vi "Save_dialogue_Q.vi"(5 "Номер образца":i32, 7 "Интеграл":dbl, 8 "0 level":bool, 9 "1 level":bool, 10 "Мощность":dbl, 11 "Амплитуда":dbl) -> (0 "OK Button 2":bool, 1 "stop 2":bool, 2 "Название 2":string, 3 "Путь 2":path)   [LabVIEW 2013]
panel:
  in  "Путь к файлу 0 уровень":path=path "d:/mech/LVPROG/1642RK2U_2port/Oscillograms/0 Level"
  in  "Путь к файлу 1 уровень":path=path "d:/mech/LVPROG/1642RK2U_2port/Oscillograms/1 Level"
  in  "Номер образца":string="1"
  in  "stop":bool
  in  "OK Button":bool
  in  "Мощность дозы":string="0,0E+0"
  in  "Путь к файлу имп.реакций":path=path "d:/mech/LVPROG/1642RK2U_2port/Oscillograms/Imp_reaction"
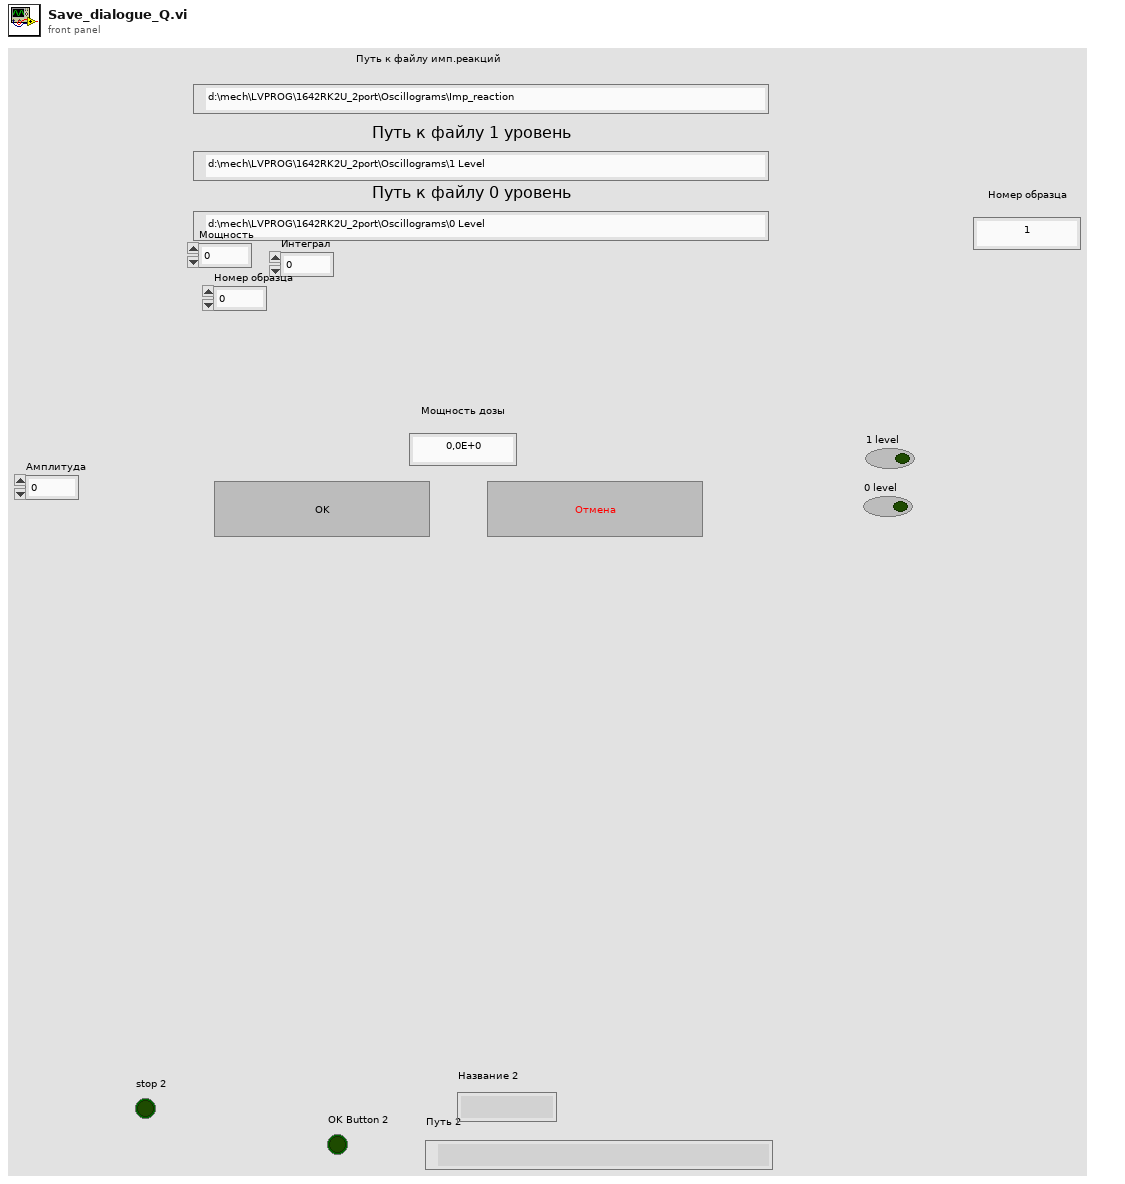
[diagram p1: front panel]
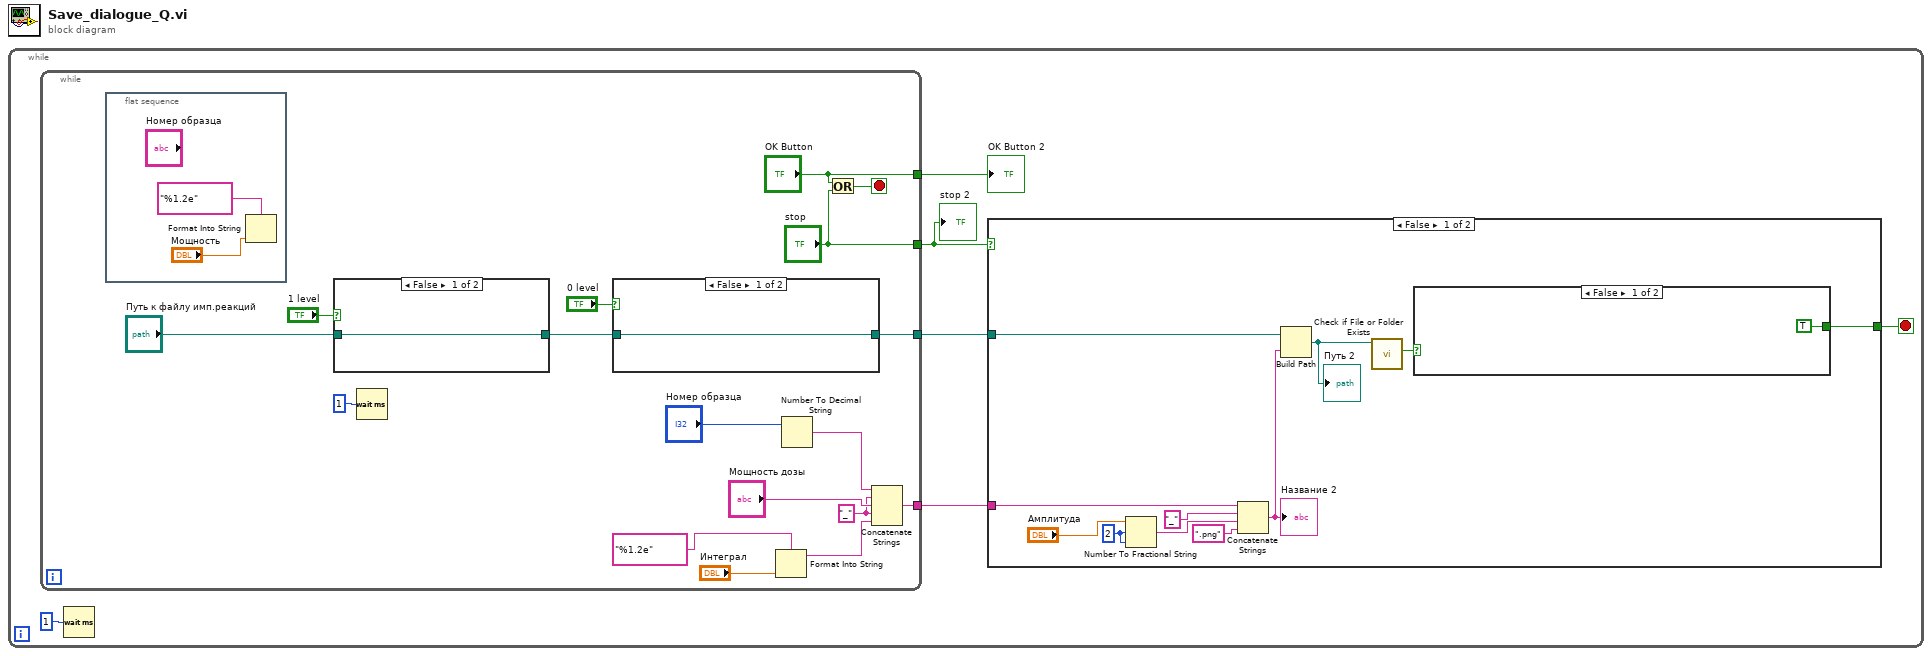
[diagram p0: block diagram]
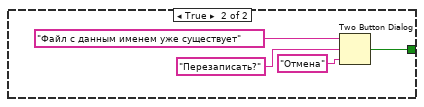
[diagram p2: hidden frame]
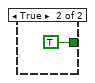
[diagram p3: hidden frame]
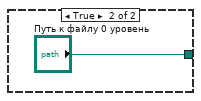
[diagram p4: hidden frame]
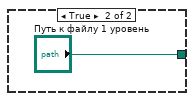
[diagram p5: hidden frame]
diagram:
  n1 = while {
    stop <- w3 stop-if-true
    n2 = while {
      tunnel: [w36] -> w2
      tunnel: ["OK Button"] -> w6
      tunnel: ["stop"] -> w4
      tunnel: [w31] -> w1
      stop <- w40 stop-if-true
      w25 = "_" ("element")
      n3 = flat-sequence {
        frame #0 {
          n4 = Format Into String(format string="%1.2e", "Мощность") -> ()  [unwired: 2 in, 2 out]
        }
      }
      n5 = case shown="False" "1 level" {
        tunnel: [w45 "Путь к файлу 1 уровень"] -> w32
        tunnel: "Путь к файлу имп.реакций" -> [w45 _]
        frame False {
        }
        frame True {
        }
      }
      n6 = Wait (ms)(milliseconds to wait=u32 1) -> ()  [unwired: 1 out]
      n7 = case shown="False" "0 level" {
        tunnel: w32 -> [w43 _]
        tunnel: [w43 "Путь к файлу 0 уровень"] -> w31
        frame False {
        }
        frame True {
        }
      }
      n8 = Format Into String(format string="%1.2e", "Интеграл") -> (resulting string=w24:string)  [unwired: 2 in, 1 out]
      n9 = Number To Decimal String(number="Номер образца") -> (decimal integer string=w30:string)  [unwired: 1 in]
      n10 = Or(x="OK Button", y="stop") -> (x .or. y?=w40:bool)
      n11 = Concatenate Strings(w30, w25, "Мощность дозы", w25, w24) -> (w36:string)
    }
    "OK Button 2" <- w6
    "stop 2" <- w4
    n12 = Wait (ms)(milliseconds to wait=u32 1) -> ()  [unwired: 1 out]
    n13 = case shown="False" w4 {
      tunnel: [w15 TRUE] -> w3
      tunnel: w2 -> [w17 _]
      tunnel: w1 -> [w10 _]
      frame False {
        w7 = i16 2 ("width (-)")
        n14 = Number To Fractional String(number="Амплитуда", width (-)=w7, precision (6)=w7) -> (F-format string=w9:string)  [unwired: 1 in]
        n15 = Concatenate Strings(w17, "_" ("element"), w9, ".png" ("element")) -> (w11:string)
        "Название 2" <- w11
        n16 = Build Path(base path=w10, name or relative path=w11) -> (appended path=w14:path)
        "Путь 2" <- w14
        n17 = call <vilib>:"Check if File or Folder Exists.vi"("path"=w14) -> ("file or folder exists?"=w16:bool)  [unwired: 8 in, 2 out]
        n18 = case shown="False" w16 {
          tunnel: [TRUE w19] -> w15
          frame False {
          }
          frame True {
            n19 = Two Button Dialog(message="Файл с данным именем уже существует", 1:"Отмена" ("F button name (\"Cancel\")"), 2:"Перезаписать?" ("T button name (\"OK\")")) -> (T button?=w19:bool)
          }
        }
      }
      frame True {
      }
    }
  }
